vi "Set Path.vi"(8 "error in (no error)":errorcluster, 10 "Path":string, 11 "URI in":refnum<class "URI.lvclass">) -> (0 "error out":errorcluster, 3 "URI out":refnum<class "URI.lvclass">)   [LabVIEW 2020, in "IO.lvlib" / "URI.lvclass"]
uses:
  URI.lvclass
  URI.lvclass/URI.ctl
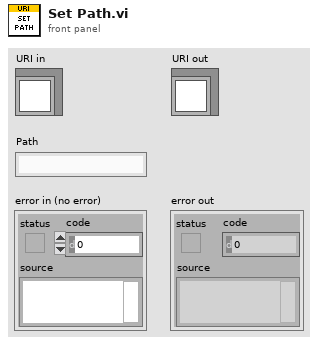
[diagram p1: front panel]
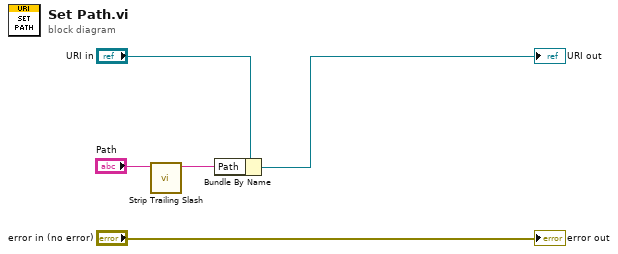
[diagram p0: block diagram]
diagram:
  n1 = call "Strip Trailing Slash.vi"("Path in"="Path") -> ("Path out"=w1:string)  [unwired: 10 in]
  n2 = Bundle By Name(cluster="URI in", "Path"=w1) -> (→"URI out":refnum<class "URI.lvclass">)
  "error out" <- "error in (no error)"
